vi "FIR Filter with I.C. (DBL).vi"(6 "Initial X Conditions":dbl[](array[numeric]), 7 "FIR Coefficients":dbl[](array[numeric]), 10 "X":dbl[](array[numeric])) -> (0 "Final X Conditions":dbl[](array[numeric]), 2 "error":i32, 3 "Filtered X":dbl[](array[numeric]))   [LabVIEW 2020, in "NI_AALBase.lvlib"]
doc: "Filters the input sequence <B>X</B> using the direct-form FIR filter specified by <B>FIR Coefficients</B>. You can use this VI to process blocks of continuous data. Wire data to the <B>X</B> input to determine the polymorphic instance to use or manually select the instance."
uses:
  NI_AALBase.lvlib
  <resource>/lvanlys.dll
panel:
  # "FIR Filter with I.C."
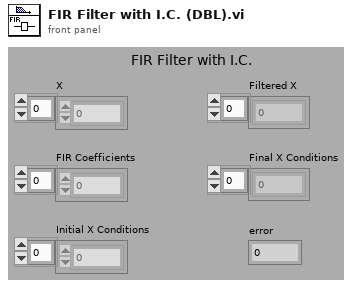
[diagram p1: front panel]
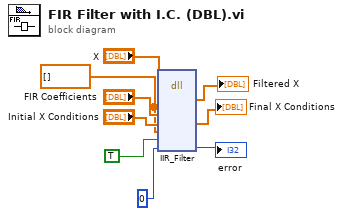
[diagram p0: block diagram]
diagram:
  w1 = dbl[] [] ("Reverse Coefficients")
  n1 = dll-call lib="C:/Program Files (x86)/National Instruments/LabVIEW 2020/resource/lvanlys.*" fn="IIR_Filter"("X"="X", "Reverse Coefficients"=w1, "FIR Coefficients"="FIR Coefficients", "Initial X Conditions"="Initial X Conditions", "Reverse Coefficients"=w1, "output param"=TRUE, "output param"=0) -> ("X"=→"Filtered X":dbl[], "Initial X Conditions"=→"Final X Conditions":dbl[], "output param"=→"error":i32)  [unwired: 8 in, 2 out]
